vi "trackTheWhale.vi"() -> ()   [LabVIEW 2014]
uses:
  <vilib>/Instr/_visa.llb/VISA Flush IO Buffer Mask.ctl
  <vilib>/Instr/_visa.llb/VISA Configure Serial Port (Instr).vi
panel:
  out "Boolean":bool
  in  "stop":bool
  out "Distance, in 2":dbl
  out "return count 2":u32
  out "read buffer 2":string
  out "Distance, in":dbl
  out "return count":u32
  out "read buffer":string
  in  "VISA resource name":refnum<visa-resource-name>="COM3"
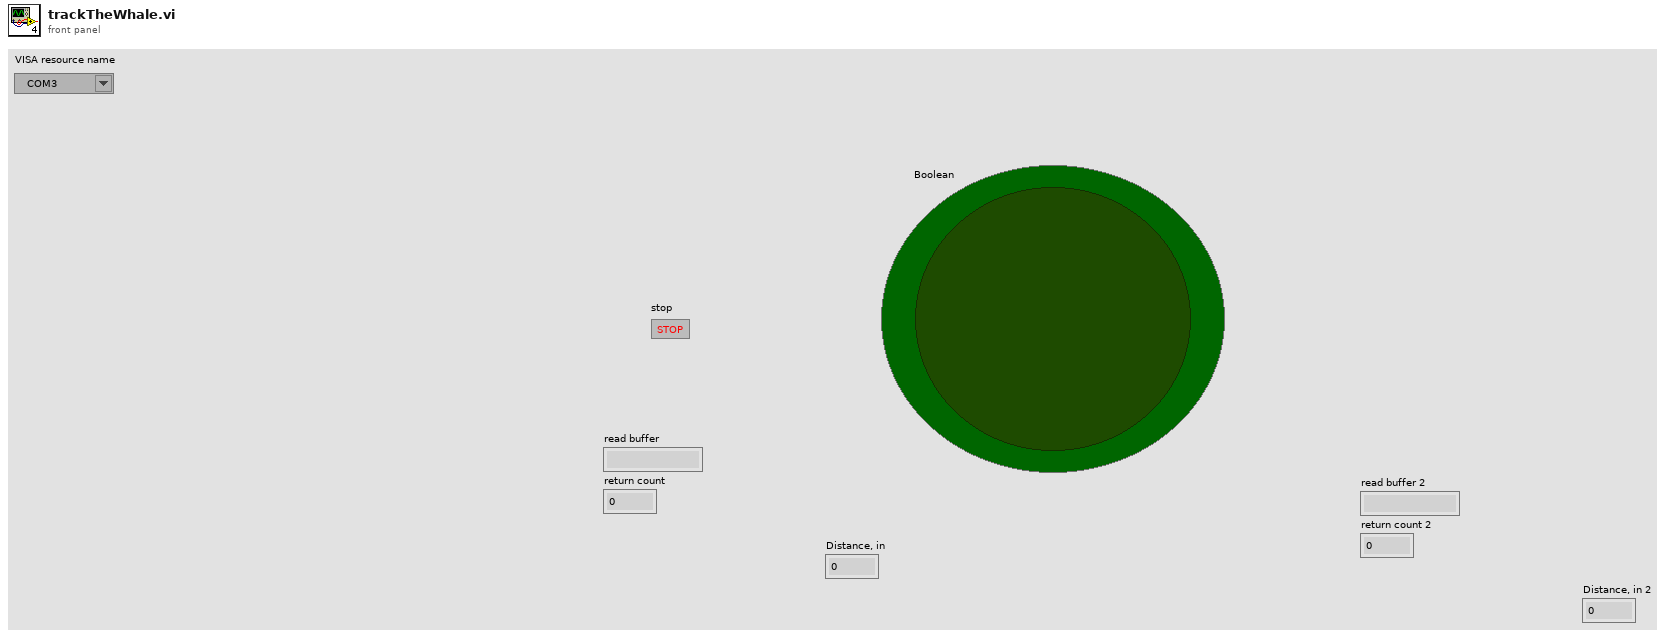
[diagram p1: front panel]
types:
  T1 = typedef "VISA Flush IO Buffer Mask.ctl" = u16
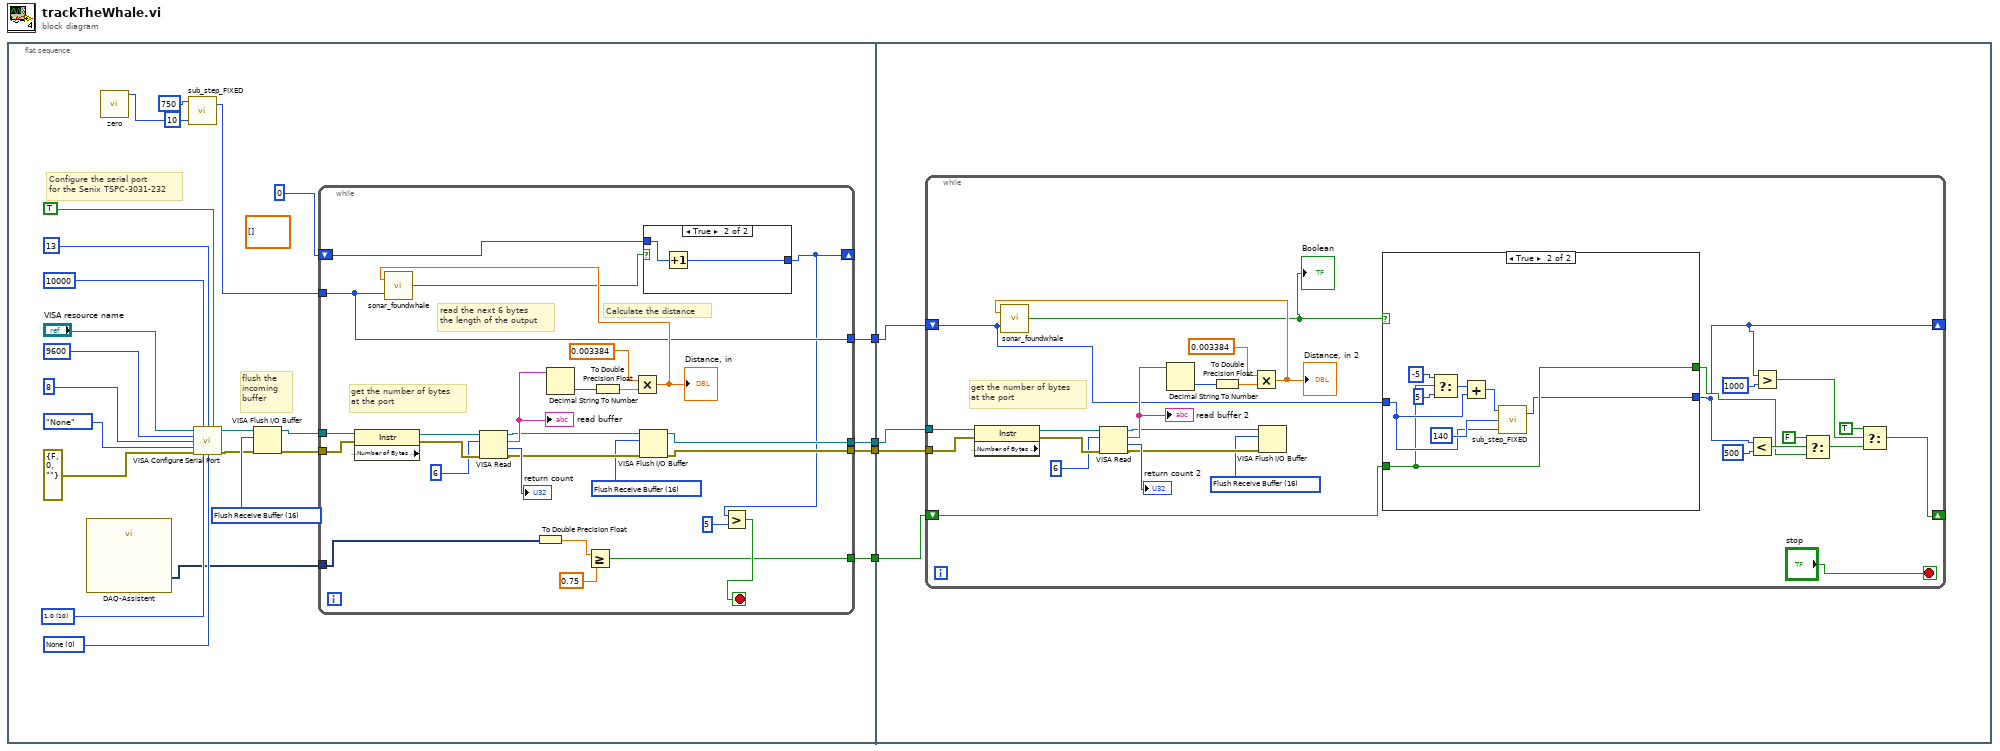
[diagram p0: block diagram]
diagram:
  n1 = flat-sequence {
    tunnel: [w11] -> w4
    tunnel: [w10] -> w3
    tunnel: [w9] -> w2
    tunnel: [w6] -> w1
    tunnel: w4 -> [w62]
    tunnel: w3 -> [w60]
    tunnel: w2 -> [w61]
    tunnel: w1 -> [w59]
    frame #0 {
      (unwired) dbl[][] []
      w16 = T1 16 items=["Flush Receive Buffer"=16, "Write Transmit Buffer to Device"=32, "Flush Receive Buffer (No I/O)"=64, "Flush Transmit Buffer"=128] ("Mask")
      w20 = u16 0 items=["None", "XON/XOFF", "RTS/CTS", "XON/XOFF & RTS/CTS", "DTR/DSR", "XON/XOFF & DTR/DSR"] ("flow control (0:none)")
      w22 = u16 10 items=["1.0"=10, "1.5"=15, "2.0"=20] ("stop bits (10: 1 bit)")
      # "flush the \nincoming \nbuffer"
      # "Configure the serial port\nfor the Senix TSPC-3031-232"
      n2 = call "DAQ-Assistent"() -> ("data"=w5:dynamicdata)  [unwired: 17 in, 2 out]
      n3 = call "zero.vi"() -> ("PositionOut"=w29:i32)  [unwired: 11 in]
      n4 = call "sub_step_FIXED.vi"("Current Position"=w29, "millisecond multiple"=u32 10, "Desired Position"=750) -> ("Position Out"=w27:i32)  [unwired: 1 in]
      n5 = call-poly "VISA Configure Serial Port"("VISA resource name"="VISA resource name", "timeout (10sec)"=u32 10000, "termination char\n(0xA = '\\n' = LF)"=u8 13 ("termination char\n(0xA = '\\n' = LF)"), "Enable Termination\nChar (T)"=TRUE ("Enable Termination\nChar (T)"), "baud rate (9600)"=u32 9600, "data bits (8)"=u16 8, "parity (0:none)"=enum16{"None", "Odd", "Even", "Mark", "Space"}."None", "error in (no error)"=errorcluster {"status"=FALSE, "code"=0, "source"=""}, "stop bits (10: 1 bit)"=w22, "flow control (0:none)"=w20) -> ("VISA resource name out"=w15:refnum<visa-resource-name>, "error out"=w14:errorcluster)  [unwired: 4 in]
      n6 = VISA Flush I/O Buffer(VISA resource name=w15, mask (16)=w16, error in (no error)=w14) -> (VISA resource name out=w13:refnum<visa-resource-name>, error out=w12:errorcluster)
      n7 = while {
        tunnel: w27 -> [w41]
        tunnel: w13 -> [w44]
        tunnel: w12 -> [w43]
        tunnel: [w41] -> w11
        tunnel: [w40] -> w10
        tunnel: [w39] -> w9
        shift-right: [w36] -> _
        shift-left: 0 -> [w37]
        tunnel: [w32] -> w6
        tunnel: w5 -> [w30]
        stop <- w35 stop-if-true
        w46 = T1 16 items=["Flush Receive Buffer"=16, "Write Transmit Buffer to Device"=32, "Flush Receive Buffer (No I/O)"=64, "Flush Transmit Buffer"=128] ("Mask")
        # "Calculate the distance"
        # "read the next 6 bytes\nthe length of the output"
        # "get the number of bytes\nat the port"
        n8 = property class="Instr" props=["Serial Settings:Number of Bytes at Serial Port"](reference=w44, error in=w43) -> (reference out=w55:refnum<visa-resource-name>, error out=w54:errorcluster)  [unwired: 1 out]
        n9 = VISA Read(VISA resource name=w55, byte count=u32 6, error in (no error)=w54) -> (VISA resource name out=w48:refnum<visa-resource-name>, read buffer=w52:string, return count=→"return count":u32, error out=w47:errorcluster)
        "read buffer" <- w52
        n10 = To Double Precision Float(number=w30) -> (double precision float=w31:dbl)
        n11 = Decimal String To Number(string=w52) -> (number=w51:i32)  [unwired: 2 in, 1 out]
        n12 = Greater Or Equal?(x=w31, y=0.75 ("byte count")) -> (x >= y?=w32:bool)
        n13 = To Double Precision Float(number=w51) -> (double precision float=w50:dbl)
        n14 = Multiply(x=0.003384, y=w50) -> (x*y=w42:dbl)
        "Distance, in" <- w42
        n15 = call "sonar_foundwhale.vi"("Current Position"=w41, "Sonar In"=w42) -> ("Found Whale"=w38:bool)
        n16 = VISA Flush I/O Buffer(VISA resource name=w48, mask (16)=w46, error in (no error)=w47) -> (VISA resource name out=w39:refnum<visa-resource-name>, error out=w40:errorcluster)
        n17 = case shown="True" w38 {
          tunnel: w37 -> [w56 w58]
          tunnel: [w56 w57] -> w36
          frame False {
          }
          frame True {
            n18 = Increment(x=w58) -> (x+1=w57:i32)
          }
        }
        n19 = Greater?(x=w36, y=5) -> (0:w35:bool)
      }
    }
    frame #1 {
      n20 = while {
        shift-right: [w66] -> _
        shift-left: w59 -> [w77]
        shift-right: [w64] -> _
        shift-left: w62 -> [w78]
        tunnel: w61 -> [w75]
        tunnel: w60 -> [w74]
        stop <- "stop" stop-if-true
        w82 = T1 16 items=["Flush Receive Buffer"=16, "Write Transmit Buffer to Device"=32, "Flush Receive Buffer (No I/O)"=64, "Flush Transmit Buffer"=128] ("Mask")
        # "get the number of bytes\nat the port"
        n21 = property class="Instr" props=["Serial Settings:Number of Bytes at Serial Port"](reference=w75, error in=w74) -> (reference out=w90:refnum<visa-resource-name>, error out=w89:errorcluster)  [unwired: 1 out]
        n22 = VISA Read(VISA resource name=w90, byte count=u32 6, error in (no error)=w89) -> (VISA resource name out=w84:refnum<visa-resource-name>, read buffer=w87:string, return count=→"return count 2":u32, error out=w83:errorcluster)
        "read buffer 2" <- w87
        n23 = Decimal String To Number(string=w87) -> (number=w86:i32)  [unwired: 2 in, 1 out]
        n24 = To Double Precision Float(number=w86) -> (double precision float=w85:dbl)
        n25 = Multiply(x=0.003384, y=w85) -> (x*y=w79:dbl)
        "Distance, in 2" <- w79
        n26 = call "sonar_foundwhale.vi"("Current Position"=w78, "Sonar In"=w79) -> ("Found Whale"=w63:bool)
        "Boolean" <- w63
        n27 = VISA Flush I/O Buffer(VISA resource name=w84, mask (16)=w82, error in (no error)=w83) -> ()  [unwired: 2 out]
        n28 = case shown="True" w63 {
          tunnel: w78 -> [w91 w95]
          tunnel: [w92 w94] -> w65
          tunnel: w77 -> [w92 w94]
          tunnel: [w91 w93] -> w64
          frame False {
          }
          frame True {
            n29 = Select(t=-5 ("byte count"), s=w94, f=5 ("byte count")) -> (s? t:f=w99:i32)
            n30 = Add(x=w99, y=w95) -> (x+y=w96:i32)
            n31 = call "sub_step_FIXED.vi"("Current Position"=w95, "millisecond multiple"=u32 140, "Desired Position"=w96) -> ("Position Out"=w93:i32)  [unwired: 1 in]
          }
        }
        n32 = Less?(x=w64, y=500 ("byte count")) -> (x < y?=w70:bool)
        n33 = Greater?(x=w64, y=1000 ("byte count")) -> (0:w71:bool)
        n34 = Select(t=FALSE, s=w70, f=w65) -> (s? t:f=w69:bool)
        n35 = Select(t=TRUE, s=w71, f=w69) -> (s? t:f=w66:bool)
      }
    }
  }
